vi "test2.vi"() -> ()   [LabVIEW 2021]
uses:
  Child.lvclass
  Parent/Parent.lvclass
panel:
  out "message":string="Parent Static  VI"
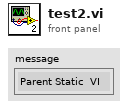
[diagram p1: front panel]
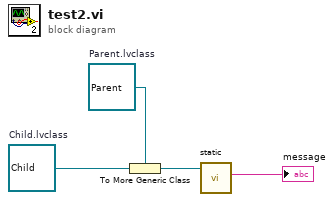
[diagram p0: block diagram]
diagram:
  w4 = refnum<class "Parent.lvclass"> refnum  # Parent.lvclass
  w3 = refnum<class "Child.lvclass"> refnum  # Child.lvclass
  n1 = To More Generic Class(target class=w4, reference=w3) -> (generic class reference=w2:refnum<class "Parent.lvclass">)
  n2 = call "static.vi"("parent in"=w2) -> ("message"=→"message":string)  [unwired: 8 in, 2 out]
